vi "Modify Numeric Rep in VI (Scalar).vi"(8 "error in":errorcluster, 10 "Modify Numeric Representation Param":T1, 11 "Original VI":path=path "C:/Users/OneEd/OneDrive/Desktop/MicroPort Job/CTDB/src/db_script/DB Select Template.vi") -> (0 "error out":errorcluster, 3 "Save as out":path=path "C:/Users/OneEd/OneDrive/Desktop/MicroPort Job/CTDB/src/db_script/DB Select Template.vi")   [LabVIEW 2021, in "EDT VI Script.lvlib"]
uses:
  EDT VI Script.lvlib
  Modify Numeric Representation Param.ctl
  <vilib>/numeric/LVNumericRepresentation.ctl
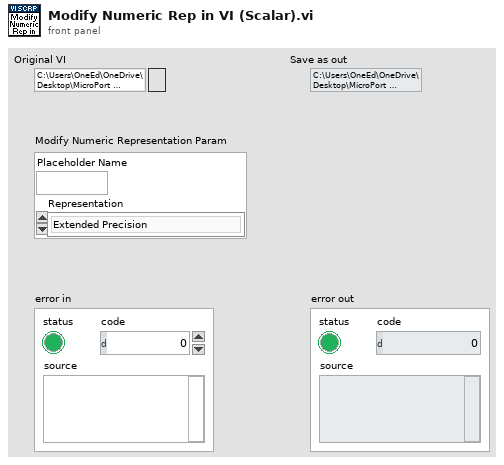
[diagram p1: front panel]
types:
  T1 = typedef "EDT VI Script.lvlib/Modify Numeric Representation Param.ctl" = cluster{"Placeholder Name":string, "Numeric Representation":T2}
  T2 = typedef "LVNumericRepresentation.ctl" = enum32{"Extended Precision", "Double Precision", "Single Precision", "Long", "Word", "Byte", "Unsigned Long", "Unsigned Word", "Unsigned Byte", "Complex Extended", "Complex Double", "Complex Single", "Quad", "Unsigned Quad", "Fixed-Point"}
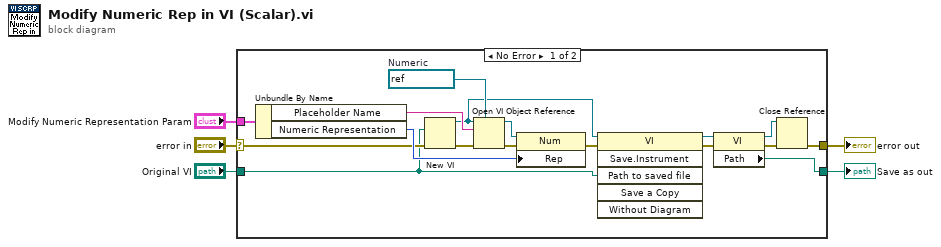
[diagram p0: block diagram]
diagram:
  n1 = case shown="No Error" "error in" {
    selector: "error in" -> [w16 w24]
    tunnel: [w6 w24] -> w4
    tunnel: "Modify Numeric Representation Param" -> [w22 _]
    tunnel: "Original VI" -> [w9 w23]
    tunnel: [w7 w23] -> w1
    frame No Error {
      w19 = refnum<vi> refnum  # Numeric
      n2 = Unbundle By Name(w22) -> ("Placeholder Name"=w21:string, "Numeric Representation"=w18:T2)
      n3 = New VI(8:w16, 10:w9) -> (0:w15:errorcluster, 3:w8:refnum<vi>)  [unwired: 5 in]
      n4 = Open VI Object Reference(7:w19, 8:w15, 10:w21, 11:w8) -> (0:w20:errorcluster, 3:w17:refnum<vi>)
      n5 = property class="Num"(reference=w17, error in=w20, "Rep"=w18) -> (error out=w10:errorcluster)  [unwired: 1 out]
      n6 = invoke class="VI" method="Save.Instrument"(reference=w8, error in=w10, "Path to saved file"=w9) -> (reference out=w12:refnum<vi>, error out=w11:errorcluster)  [unwired: 3 in, 4 out]
      n7 = property class="VI"(reference=w12, error in=w11) -> (reference out=w14:refnum<vi>, error out=w13:errorcluster, "Path"=w7:path)
      n8 = Close Reference(reference=w14, error in (no error)=w13) -> (error out=w6:errorcluster)
    }
    frame Error {
    }
  }
  "error out" <- w4
  "Save as out" <- w1
